vi "Write_tcpListenerID.vi"(8 "error in (no error)":errorcluster, 10 "tcpListenerID":refnum<k5>, 11 "tcpServer in":refnum<class "TcpServer.lvclass">) -> (0 "error out":errorcluster, 3 "tcpServer out":refnum<class "TcpServer.lvclass">)   [LabVIEW 2018, in "TcpServer.lvclass"]
doc: "Write the TCP Listener ID after the TCP Create Listener function is executed."
uses:
  TcpServer.lvclass
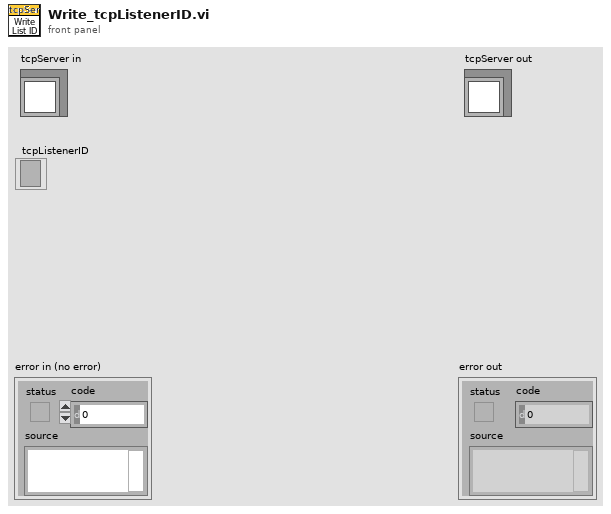
[diagram p1: front panel]
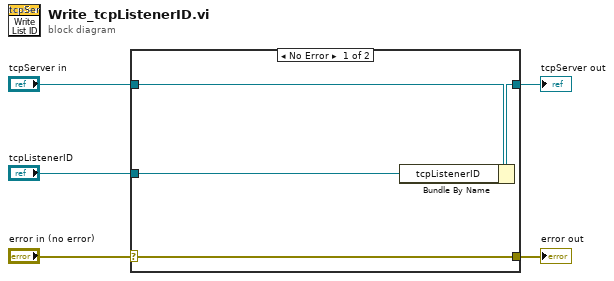
[diagram p0: block diagram]
diagram:
  n1 = case shown="No Error" "error in (no error)" {
    selector: "error in (no error)" -> [w9 w10]
    tunnel: [w9 w10] -> w4
    tunnel: [w7 w11] -> w2
    tunnel: "tcpServer in" -> [w8 w11]
    tunnel: "tcpListenerID" -> [w6 _]
    frame No Error {
      n2 = Bundle By Name(cluster=w8, "tcpListenerID"=w6) -> (w7:refnum<class "TcpServer.lvclass">)
    }
    frame Error {
    }
  }
  "error out" <- w4
  "tcpServer out" <- w2
